vi "Lab Panel V4.83.vi"() -> ()   [LabVIEW 2013] (continued)
                  tunnel: w884 -> [_ w917]
                  tunnel: [w889 w916] -> w883
                  frame False {
                    # "stop test"
                    n577 = stacked-sequence {
                      tunnel: w890 -> [w899 _]
                      tunnel: [w891 _] -> w889
                      frame #0 {
                        n578 = local read "DISP LAB02-2"() -> (w898:T4)
                        n579 = Unbundle(w898) -> ("CYCLE"=w896:dbl, "MINS"=w897:dbl)  [unwired: 1 out]
                        n580 = case shown="\"CYCLE TEST\"" w899 {
                          tunnel: w897 -> [_ _ w906]
                          tunnel: w896 -> [w904 w905 _]
                          tunnel: [w904 w905 w906] -> w895
                          frame "CHART TEST", Default {
                          }
                          frame "CYCLE TEST" {
                          }
                          frame "T-RISE TEST" {
                          }
                        }
                        n581 = local read "TDMS LAB02-2"() -> (w903:refnum<k34>)
                        n582 = Build Array("STOPPED") -> (w900:string[])
                        n583 = Build Array(w895) -> (w894:dbl[])
                        n584 = TDMS Write(0:w903, 5:"TEST RESULT", 7:w900, 9:w894) -> (4:w892:refnum<k34>, 15:w893:errorcluster)  [unwired: 2 in, 2 out]
                        n585 = TDMS Close(8:w893, 11:w892) -> (0:w891:errorcluster)  [unwired: 1 out]
                      }
                      frame #1 {
                        n586 = local read "DISP LAB02-2"() -> (w910:T4)
                        n587 = stacked-sequence {
                          tunnel: "LAB02-2" -> [w912 w914]
                          frame #0 {
                            n588 = call "sub vi - defrag tdms v1.vi"("panel id"=w912) -> ("error out"=w911:errorcluster)  [unwired: 10 in]
                            n589 = local write "data file error"(w911) -> ()
                          }
                          frame #1 {
                            n590 = call "Save data file to network drive v2.vi"("panel id"=w914) -> ("network file save error"=w913:errorcluster)  [unwired: 9 in, 1 out]
                            n591 = local write "RESULT LAB02-2"(FALSE) -> ()
                            n592 = local write "data file error"(w913) -> ()
                          }
                        }
                        n593 = Bundle(cluster=w910, "STATUS"="STOP") -> (w908:T4)  [unwired: 2 in]
                        n594 = local write "DISP LAB02-2"(w908) -> ()
                      }
                    }
                  }
                  frame True {
                    # "start new test and create test file"
                    n595 = stacked-sequence {
                      seq-local: [w922 _ _ _ _] -> [_ w946 _ _ _]
                      tunnel: w921 -> [w927 _ _ _ _]
                      tunnel: w920 -> [w924 _ _ _ _]
                      tunnel: w919 -> [w937 _ _ _ _]
                      tunnel: w918 -> [w930 _ _ _ _]
                      tunnel: w917 -> [w925 _ _ _ _]
                      tunnel: [_ w941 _ _ _] -> w916
                      frame #0 {
                        w923 = "\\"
                        n596 = local read "SET LAB02-2"() -> (w932:T5)
                        n597 = case shown="\"CYCLE TEST\"" w937 {
                          tunnel: ["L02-2-CHART TEST-" "L02-2-CYCLE TEST-" "L02-2-T-RISE TEST-"] -> w933
                          frame "CHART TEST", Default {
                          }
                          frame "CYCLE TEST" {
                          }
                          frame "T-RISE TEST" {
                          }
                        }
                        n598 = Unbundle(w932) -> ("DESCRIPTION"=w931:string)  [unwired: 4 out]
                        n599 = Concatenate Strings(w927, "\\", w925, w923, w924, w923) -> (w934:string)
                        n600 = String To Path(string=w934) -> (path=w936:path)
                        n601 = Concatenate Strings(w934, w933, w931, "-", w930, ".tdms") -> (w922:string)
                        n602 = Create Folder(path (use dialog)=w936) -> (error out=w935:errorcluster)  [unwired: 2 in, 2 out]
                        n603 = global write "Global 1.vi" "LAB02-2 FILE"(w922) -> ()
                        n604 = call <vilib>:"Clear Errors.vi"("error in (no error)"=w935) -> ()  [unwired: 6 in, 1 out]
                      }
                      frame #1 {
                        (unwired) FALSE
                        n605 = String To Path(string=w946) -> (path=w942:path)
                        n606 = TDMS Open(6:FALSE, 10:T18."create or replace" ("operation (0:open)"), 11:w942) -> (0:w941:errorcluster, 3:→"TDMS LAB02-2":refnum<k34>)  [unwired: 4 in]
                      }
                      frame #2 {
                        n607 = local read "SET LAB02-2"() -> (w952:T5)
                        n608 = local read "TDMS LAB02-2"() -> (w963:refnum<k34>)
                        n609 = Build Array("Testers Name", "Description", "Set Test Cycles", "T-Rise minutes", "T-Rise Deg C") -> (w953:string[])
                        n610 = Unbundle(w952) -> ("NAME"=w951:string, "DESCRIPTION"=w950:string, "CYCLES"=w949:dbl, "T-RISE mins"=w948:dbl, "T-RISE deg C"=w947:dbl)
                        n611 = Number To Decimal String(number=w949) -> (decimal integer string=w962:string)  [unwired: 1 in]
                        n612 = Number To Decimal String(number=w948) -> (decimal integer string=w961:string)  [unwired: 1 in]
                        n613 = Number To Decimal String(number=w947) -> (decimal integer string=w960:string)  [unwired: 1 in]
                        n614 = Build Array(w951, w950, w962, w961, w960) -> (w959:string[])
                        n615 = TDMS Set Properties(5:w959, 7:w953, 11:w963) -> ()  [unwired: 3 in, 4 out]
                      }
                      frame #3 {
                        w965 = 0.0
                        n616 = local read "DISP LAB02-2"() -> (w967:T4)
                        n617 = Bundle(cluster=w967, "CYCLE"=w965, "MINS"=w965, "STATUS"="RUN") -> (w966:T4)
                        n618 = local write "DISP LAB02-2"(w966) -> ()
                      }
                      frame #4 {
                        n619 = local read "SIG LAB02-2"() -> (w970:T2)
                        n620 = local read "TEMP START LAB02-2"() -> (w972:cluster{"TL":dbl, "TN":dbl})
                        n621 = Unbundle(w970) -> ("Tmp Live"=w969:dbl, "Tmp Neut"=w968:dbl)  [unwired: 3 out]
                        n622 = Bundle(cluster=w972, "TL"=w969, "TN"=w968) -> (w971:cluster{"TL":dbl, "TN":dbl})
                        n623 = local write "TEMP START LAB02-2"(w971) -> ()
                      }
                    }
                  }
                }
              }
              event "RUN LAB03-1": Value Change {
                n624 = event-data() -> ("NewVal"=w973:bool)  [unwired: 1 in, 5 out]
                n625 = local write "run lab03-1"(w973) -> ()
                n626 = case shown="False" w973 {
                  tunnel: w979 -> [_ w1012]
                  tunnel: w978 -> [_ w1011]
                  tunnel: w976 -> [w981 w1010]
                  tunnel: w977 -> [_ w1009]
                  tunnel: w975 -> [_ w1008]
                  tunnel: [w980 w1007] -> w974
                  frame False {
                    # "stop test"
                    n627 = stacked-sequence {
                      tunnel: w981 -> [w990 _]
                      tunnel: [w982 _] -> w980
                      frame #0 {
                        n628 = local read "DISP LAB03-1"() -> (w989:T4)
                        n629 = Unbundle(w989) -> ("CYCLE"=w987:dbl, "MINS"=w988:dbl)  [unwired: 1 out]
                        n630 = case shown="\"CYCLE TEST\"" w990 {
                          tunnel: w988 -> [_ _ w997]
                          tunnel: w987 -> [w995 w996 _]
                          tunnel: [w995 w996 w997] -> w986
                          frame "CHART TEST", Default {
                          }
                          frame "CYCLE TEST" {
                          }
                          frame "T-RISE TEST" {
                          }
                        }
                        n631 = local read "TDMS LAB03-1"() -> (w994:refnum<k34>)
                        n632 = Build Array("STOPPED") -> (w991:string[])
                        n633 = Build Array(w986) -> (w985:dbl[])
                        n634 = TDMS Write(0:w994, 5:"TEST RESULT", 7:w991, 9:w985) -> (4:w983:refnum<k34>, 15:w984:errorcluster)  [unwired: 2 in, 2 out]
                        n635 = TDMS Close(8:w984, 11:w983) -> (0:w982:errorcluster)  [unwired: 1 out]
                      }
                      frame #1 {
                        n636 = local read "DISP LAB03-1"() -> (w1001:T4)
                        n637 = stacked-sequence {
                          tunnel: "LAB03-1" -> [w1003 w1005]
                          frame #0 {
                            n638 = call "sub vi - defrag tdms v1.vi"("panel id"=w1003) -> ("error out"=w1002:errorcluster)  [unwired: 10 in]
                            n639 = local write "data file error"(w1002) -> ()
                          }
                          frame #1 {
                            n640 = call "Save data file to network drive v2.vi"("panel id"=w1005) -> ("network file save error"=w1004:errorcluster)  [unwired: 9 in, 1 out]
                            n641 = local write "RESULT LAB03-1"(FALSE) -> ()
                            n642 = local write "data file error"(w1004) -> ()
                          }
                        }
                        n643 = Bundle(cluster=w1001, "STATUS"="STOP") -> (w999:T4)  [unwired: 2 in]
                        n644 = local write "DISP LAB03-1"(w999) -> ()
                      }
                    }
                  }
                  frame True {
                    # "start new test and create test file"
                    n645 = stacked-sequence {
                      seq-local: [w1013 _ _ _ _] -> [_ w1037 _ _ _]
                      tunnel: w1012 -> [w1018 _ _ _ _]
                      tunnel: w1011 -> [w1015 _ _ _ _]
                      tunnel: w1010 -> [w1028 _ _ _ _]
                      tunnel: w1009 -> [w1021 _ _ _ _]
                      tunnel: w1008 -> [w1016 _ _ _ _]
                      tunnel: [_ w1032 _ _ _] -> w1007
                      frame #0 {
                        w1014 = "\\"
                        n646 = local read "SET LAB03-1"() -> (w1023:T5)
                        n647 = case shown="\"T-RISE TEST\"" w1028 {
                          tunnel: ["L03-1-CHART TEST-" "L03-1-CYCLE TEST-" "L03-1-T-RISE TEST-"] -> w1024
                          frame "CHART TEST", Default {
                          }
                          frame "CYCLE TEST" {
                          }
                          frame "T-RISE TEST" {
                          }
                        }
                        n648 = Unbundle(w1023) -> ("DESCRIPTION"=w1022:string)  [unwired: 4 out]
                        n649 = Concatenate Strings(w1018, "\\", w1016, w1014, w1015, w1014) -> (w1025:string)
                        n650 = String To Path(string=w1025) -> (path=w1027:path)
                        n651 = Concatenate Strings(w1025, w1024, w1022, "-", w1021, ".tdms") -> (w1013:string)
                        n652 = Create Folder(path (use dialog)=w1027) -> (error out=w1026:errorcluster)  [unwired: 2 in, 2 out]
                        n653 = global write "Global 1.vi" "LAB03-1 FILE"(w1013) -> ()
                        n654 = call <vilib>:"Clear Errors.vi"("error in (no error)"=w1026) -> ()  [unwired: 6 in, 1 out]
                      }
                      frame #1 {
                        (unwired) FALSE
                        n655 = String To Path(string=w1037) -> (path=w1033:path)
                        n656 = TDMS Open(6:FALSE, 10:T18."create or replace" ("operation (0:open)"), 11:w1033) -> (0:w1032:errorcluster, 3:→"TDMS LAB03-1":refnum<k34>)  [unwired: 4 in]
                      }
                      frame #2 {
                        n657 = local read "SET LAB03-1"() -> (w1043:T5)
                        n658 = local read "TDMS LAB03-1"() -> (w1054:refnum<k34>)
                        n659 = Build Array("Testers Name", "Description", "Set Test Cycles", "T-Rise minutes", "T-Rise Deg C") -> (w1044:string[])
                        n660 = Unbundle(w1043) -> ("NAME"=w1042:string, "DESCRIPTION"=w1041:string, "CYCLES"=w1040:dbl, "T-RISE mins"=w1039:dbl, "T-RISE deg C"=w1038:dbl)
                        n661 = Number To Decimal String(number=w1040) -> (decimal integer string=w1053:string)  [unwired: 1 in]
                        n662 = Number To Decimal String(number=w1039) -> (decimal integer string=w1052:string)  [unwired: 1 in]
                        n663 = Number To Decimal String(number=w1038) -> (decimal integer string=w1051:string)  [unwired: 1 in]
                        n664 = Build Array(w1042, w1041, w1053, w1052, w1051) -> (w1050:string[])
                        n665 = TDMS Set Properties(5:w1050, 7:w1044, 11:w1054) -> ()  [unwired: 3 in, 4 out]
                      }
                      frame #3 {
                        w1056 = 0.0
                        n666 = local read "DISP LAB03-1"() -> (w1058:T4)
                        n667 = Bundle(cluster=w1058, "CYCLE"=w1056, "MINS"=w1056, "STATUS"="RUN") -> (w1057:T4)
                        n668 = local write "DISP LAB03-1"(w1057) -> ()
                      }
                      frame #4 {
                        n669 = local read "SIG LAB03-1"() -> (w1061:T2)
                        n670 = local read "TEMP START LAB03-1"() -> (w1063:cluster{"TL":dbl, "TN":dbl})
                        n671 = Unbundle(w1061) -> ("Tmp Live"=w1060:dbl, "Tmp Neut"=w1059:dbl)  [unwired: 3 out]
                        n672 = Bundle(cluster=w1063, "TL"=w1060, "TN"=w1059) -> (w1062:cluster{"TL":dbl, "TN":dbl})
                        n673 = local write "TEMP START LAB03-1"(w1062) -> ()
                      }
                    }
                  }
                }
              }
              event "RUN LAB03-2": Value Change {
                n674 = event-data() -> ("NewVal"=w1064:bool)  [unwired: 1 in, 5 out]
                n675 = local write "run lab03-2"(w1064) -> ()
                n676 = case shown="True" w1064 {
                  tunnel: w1070 -> [_ w1103]
                  tunnel: w1069 -> [_ w1102]
                  tunnel: w1067 -> [w1072 w1101]
                  tunnel: w1068 -> [_ w1100]
                  tunnel: w1066 -> [_ w1099]
                  tunnel: [w1071 w1098] -> w1065
                  frame False {
                    # "stop test"
                    n677 = stacked-sequence {
                      tunnel: w1072 -> [w1081 _]
                      tunnel: [w1073 _] -> w1071
                      frame #0 {
                        n678 = local read "DISP LAB03-2"() -> (w1080:T4)
                        n679 = Unbundle(w1080) -> ("CYCLE"=w1078:dbl, "MINS"=w1079:dbl)  [unwired: 1 out]
                        n680 = case shown="\"CYCLE TEST\"" w1081 {
                          tunnel: w1079 -> [_ _ w1088]
                          tunnel: w1078 -> [w1086 w1087 _]
                          tunnel: [w1086 w1087 w1088] -> w1077
                          frame "CHART TEST", Default {
                          }
                          frame "CYCLE TEST" {
                          }
                          frame "T-RISE TEST" {
                          }
                        }
                        n681 = local read "TDMS LAB03-2"() -> (w1085:refnum<k34>)
                        n682 = Build Array("STOPPED") -> (w1082:string[])
                        n683 = Build Array(w1077) -> (w1076:dbl[])
                        n684 = TDMS Write(0:w1085, 5:"TEST RESULT", 7:w1082, 9:w1076) -> (4:w1074:refnum<k34>, 15:w1075:errorcluster)  [unwired: 2 in, 2 out]
                        n685 = TDMS Close(8:w1075, 11:w1074) -> (0:w1073:errorcluster)  [unwired: 1 out]
                      }
                      frame #1 {
                        n686 = local read "DISP LAB03-2"() -> (w1092:T4)
                        n687 = stacked-sequence {
                          tunnel: "LAB03-2" -> [w1094 w1096]
                          frame #0 {
                            n688 = call "sub vi - defrag tdms v1.vi"("panel id"=w1094) -> ("error out"=w1093:errorcluster)  [unwired: 10 in]
                            n689 = local write "data file error"(w1093) -> ()
                          }
                          frame #1 {
                            n690 = call "Save data file to network drive v2.vi"("panel id"=w1096) -> ("network file save error"=w1095:errorcluster)  [unwired: 9 in, 1 out]
                            n691 = local write "RESULT LAB03-2"(FALSE) -> ()
                            n692 = local write "data file error"(w1095) -> ()
                          }
                        }
                        n693 = Bundle(cluster=w1092, "STATUS"="STOP") -> (w1090:T4)  [unwired: 2 in]
                        n694 = local write "DISP LAB03-2"(w1090) -> ()
                      }
                    }
                  }
                  frame True {
                    # "start new test and create test file"
                    n695 = stacked-sequence {
                      seq-local: [w1104 _ _ _ _] -> [_ w1128 _ _ _]
                      tunnel: w1103 -> [w1109 _ _ _ _]
                      tunnel: w1102 -> [w1106 _ _ _ _]
                      tunnel: w1101 -> [w1119 _ _ _ _]
                      tunnel: w1100 -> [w1112 _ _ _ _]
                      tunnel: w1099 -> [w1107 _ _ _ _]
                      tunnel: [_ w1123 _ _ _] -> w1098
                      frame #0 {
                        w1105 = "\\"
                        n696 = local read "SET LAB03-2"() -> (w1114:T5)
                        n697 = case shown="\"T-RISE TEST\"" w1119 {
                          tunnel: ["L03-2-CHART TEST-" "L03-2-CYCLE TEST-" "L03-2-T-RISE TEST-"] -> w1115
                          frame "CHART TEST", Default {
                          }
                          frame "CYCLE TEST" {
                          }
                          frame "T-RISE TEST" {
                          }
                        }
                        n698 = Unbundle(w1114) -> ("DESCRIPTION"=w1113:string)  [unwired: 4 out]
                        n699 = Concatenate Strings(w1109, "\\", w1107, w1105, w1106, w1105) -> (w1116:string)
                        n700 = String To Path(string=w1116) -> (path=w1118:path)
                        n701 = Concatenate Strings(w1116, w1115, w1113, "-", w1112, ".tdms") -> (w1104:string)
                        n702 = Create Folder(path (use dialog)=w1118) -> (error out=w1117:errorcluster)  [unwired: 2 in, 2 out]
                        n703 = global write "Global 1.vi" "LAB03-2 FILE"(w1104) -> ()
                        n704 = call <vilib>:"Clear Errors.vi"("error in (no error)"=w1117) -> ()  [unwired: 6 in, 1 out]
                      }
                      frame #1 {
                        (unwired) FALSE
                        n705 = String To Path(string=w1128) -> (path=w1124:path)
                        n706 = TDMS Open(6:FALSE, 10:T18."create or replace" ("operation (0:open)"), 11:w1124) -> (0:w1123:errorcluster, 3:→"TDMS LAB03-2":refnum<k34>)  [unwired: 4 in]
                      }
                      frame #2 {
                        n707 = local read "SET LAB03-2"() -> (w1134:T5)
                        n708 = local read "TDMS LAB03-2"() -> (w1145:refnum<k34>)
                        n709 = Build Array("Testers Name", "Description", "Set Test Cycles", "T-Rise minutes", "T-Rise Deg C") -> (w1135:string[])
                        n710 = Unbundle(w1134) -> ("NAME"=w1133:string, "DESCRIPTION"=w1132:string, "CYCLES"=w1131:dbl, "T-RISE mins"=w1130:dbl, "T-RISE deg C"=w1129:dbl)
                        n711 = Number To Decimal String(number=w1131) -> (decimal integer string=w1144:string)  [unwired: 1 in]
                        n712 = Number To Decimal String(number=w1130) -> (decimal integer string=w1143:string)  [unwired: 1 in]
                        n713 = Number To Decimal String(number=w1129) -> (decimal integer string=w1142:string)  [unwired: 1 in]
                        n714 = Build Array(w1133, w1132, w1144, w1143, w1142) -> (w1141:string[])
                        n715 = TDMS Set Properties(5:w1141, 7:w1135, 11:w1145) -> ()  [unwired: 3 in, 4 out]
                      }
                      frame #3 {
                        w1147 = 0.0
                        n716 = local read "DISP LAB03-2"() -> (w1149:T4)
                        n717 = Bundle(cluster=w1149, "CYCLE"=w1147, "MINS"=w1147, "STATUS"="RUN") -> (w1148:T4)
                        n718 = local write "DISP LAB03-2"(w1148) -> ()
                      }
                      frame #4 {
                        n719 = local read "SIG LAB03-2"() -> (w1152:T2)
                        n720 = local read "TEMP START LAB03-2"() -> (w1154:cluster{"TL":dbl, "TN":dbl})
                        n721 = Unbundle(w1152) -> ("Tmp Live"=w1151:dbl, "Tmp Neut"=w1150:dbl)  [unwired: 3 out]
                        n722 = Bundle(cluster=w1154, "TL"=w1151, "TN"=w1150) -> (w1153:cluster{"TL":dbl, "TN":dbl})
                        n723 = local write "TEMP START LAB03-2"(w1153) -> ()
                      }
                    }
                  }
                }
              }
              event "RUN LAB04-1": Value Change {
                n724 = event-data() -> ("NewVal"=w1155:bool)  [unwired: 1 in, 5 out]
                n725 = local write "run lab04-1"(w1155) -> ()
                n726 = case shown="True" w1155 {
                  tunnel: w1161 -> [_ w1194]
                  tunnel: w1160 -> [_ w1193]
                  tunnel: w1158 -> [w1163 w1192]
                  tunnel: w1159 -> [_ w1191]
                  tunnel: w1157 -> [_ w1190]
                  tunnel: [w1162 w1189] -> w1156
                  frame False {
                    # "stop test"
                    n727 = stacked-sequence {
                      tunnel: w1163 -> [w1172 _]
                      tunnel: [w1164 _] -> w1162
                      frame #0 {
                        n728 = local read "DISP LAB04-1"() -> (w1171:T4)
                        n729 = Unbundle(w1171) -> ("CYCLE"=w1169:dbl, "MINS"=w1170:dbl)  [unwired: 1 out]
                        n730 = case shown="\"CYCLE TEST\"" w1172 {
                          tunnel: w1170 -> [_ _ w1179]
                          tunnel: w1169 -> [w1177 w1178 _]
                          tunnel: [w1177 w1178 w1179] -> w1168
                          frame "CHART TEST", Default {
                          }
                          frame "CYCLE TEST" {
                          }
                          frame "T-RISE TEST" {
                          }
                        }
                        n731 = local read "TDMS LAB04-1"() -> (w1176:refnum<k34>)
                        n732 = Build Array("STOPPED") -> (w1173:string[])
                        n733 = Build Array(w1168) -> (w1167:dbl[])
                        n734 = TDMS Write(0:w1176, 5:"TEST RESULT", 7:w1173, 9:w1167) -> (4:w1165:refnum<k34>, 15:w1166:errorcluster)  [unwired: 2 in, 2 out]
                        n735 = TDMS Close(8:w1166, 11:w1165) -> (0:w1164:errorcluster)  [unwired: 1 out]
                      }
                      frame #1 {
                        n736 = local read "DISP LAB04-1"() -> (w1183:T4)
                        n737 = stacked-sequence {
                          tunnel: "LAB04-1" -> [w1185 w1187]
                          frame #0 {
                            n738 = call "sub vi - defrag tdms v1.vi"("panel id"=w1185) -> ("error out"=w1184:errorcluster)  [unwired: 10 in]
                            n739 = local write "data file error"(w1184) -> ()
                          }
                          frame #1 {
                            n740 = call "Save data file to network drive v2.vi"("panel id"=w1187) -> ("network file save error"=w1186:errorcluster)  [unwired: 9 in, 1 out]
                            n741 = local write "RESULT LAB04-1"(FALSE) -> ()
                            n742 = local write "data file error"(w1186) -> ()
                          }
                        }
                        n743 = Bundle(cluster=w1183, "STATUS"="STOP") -> (w1181:T4)  [unwired: 2 in]
                        n744 = local write "DISP LAB04-1"(w1181) -> ()
                      }
                    }
                  }
                  frame True {
                    # "start new test and create test file"
                    n745 = stacked-sequence {
                      seq-local: [w1195 _ _ _ _] -> [_ w1219 _ _ _]
                      tunnel: w1194 -> [w1200 _ _ _ _]
                      tunnel: w1193 -> [w1196 _ _ _ _]
                      tunnel: w1192 -> [w1210 _ _ _ _]
                      tunnel: w1191 -> [w1203 _ _ _ _]
                      tunnel: w1190 -> [w1198 _ _ _ _]
                      tunnel: [_ w1214 _ _ _] -> w1189
                      frame #0 {
                        w1197 = "\\"
                        n746 = local read "SET LAB04-1"() -> (w1205:T5)
                        n747 = case shown="\"CYCLE TEST\"" w1210 {
                          tunnel: ["L04-1-CHART TEST-" "L04-1-CYCLE TEST-" "L04-1-T-RISE TEST-"] -> w1206
                          frame "CHART TEST", Default {
                          }
                          frame "CYCLE TEST" {
                          }
                          frame "T-RISE TEST" {
                          }
                        }
                        n748 = Unbundle(w1205) -> ("DESCRIPTION"=w1204:string)  [unwired: 4 out]
                        n749 = Concatenate Strings(w1200, "\\", w1198, w1197, w1196, w1197) -> (w1207:string)
                        n750 = String To Path(string=w1207) -> (path=w1209:path)
                        n751 = Concatenate Strings(w1207, w1206, w1204, "-", w1203, ".tdms") -> (w1195:string)
                        n752 = Create Folder(path (use dialog)=w1209) -> (error out=w1208:errorcluster)  [unwired: 2 in, 2 out]
                        n753 = global write "Global 1.vi" "LAB04-1 FILE"(w1195) -> ()
                        n754 = call <vilib>:"Clear Errors.vi"("error in (no error)"=w1208) -> ()  [unwired: 6 in, 1 out]
                      }
                      frame #1 {
                        (unwired) FALSE
                        n755 = String To Path(string=w1219) -> (path=w1215:path)
                        n756 = TDMS Open(6:FALSE, 10:T18."create or replace" ("operation (0:open)"), 11:w1215) -> (0:w1214:errorcluster, 3:→"TDMS LAB04-1":refnum<k34>)  [unwired: 4 in]
                      }
                      frame #2 {
                        n757 = local read "SET LAB04-1"() -> (w1225:T5)
                        n758 = local read "TDMS LAB04-1"() -> (w1236:refnum<k34>)
                        n759 = Build Array("Testers Name", "Description", "Set Test Cycles", "T-Rise minutes", "T-Rise Deg C") -> (w1226:string[])
                        n760 = Unbundle(w1225) -> ("NAME"=w1224:string, "DESCRIPTION"=w1223:string, "CYCLES"=w1222:dbl, "T-RISE mins"=w1221:dbl, "T-RISE deg C"=w1220:dbl)
                        n761 = Number To Decimal String(number=w1222) -> (decimal integer string=w1235:string)  [unwired: 1 in]
                        n762 = Number To Decimal String(number=w1221) -> (decimal integer string=w1234:string)  [unwired: 1 in]
                        n763 = Number To Decimal String(number=w1220) -> (decimal integer string=w1233:string)  [unwired: 1 in]
                        n764 = Build Array(w1224, w1223, w1235, w1234, w1233) -> (w1232:string[])
                        n765 = TDMS Set Properties(5:w1232, 7:w1226, 11:w1236) -> ()  [unwired: 3 in, 4 out]
                      }
                      frame #3 {
                        w1238 = 0.0
                        n766 = local read "DISP LAB04-1"() -> (w1240:T4)
                        n767 = Bundle(cluster=w1240, "CYCLE"=w1238, "MINS"=w1238, "STATUS"="RUN") -> (w1239:T4)
                        n768 = local write "DISP LAB04-1"(w1239) -> ()
                      }
                      frame #4 {
                        n769 = local read "SIG LAB04-1"() -> (w1243:T2)
                        n770 = local read "TEMP START LAB04-1"() -> (w1245:cluster{"TL":dbl, "TN":dbl})
                        n771 = Unbundle(w1243) -> ("Tmp Live"=w1242:dbl, "Tmp Neut"=w1241:dbl)  [unwired: 3 out]
                        n772 = Bundle(cluster=w1245, "TL"=w1242, "TN"=w1241) -> (w1244:cluster{"TL":dbl, "TN":dbl})
                        n773 = local write "TEMP START LAB04-1"(w1244) -> ()
                      }
                    }
                  }
                }
              }
              event "RUN LAB04-2": Value Change {
                n774 = event-data() -> ("NewVal"=w1246:bool)  [unwired: 1 in, 5 out]
                n775 = local write "run lab04-2"(w1246) -> ()
                n776 = case shown="True" w1246 {
                  tunnel: w1252 -> [_ w1285]
                  tunnel: w1251 -> [_ w1284]
                  tunnel: w1249 -> [w1254 w1283]
                  tunnel: w1250 -> [_ w1282]
                  tunnel: w1248 -> [_ w1281]
                  tunnel: [w1253 w1280] -> w1247
                  frame False {
                    # "stop test"
                    n777 = stacked-sequence {
                      tunnel: w1254 -> [w1263 _]
                      tunnel: [w1255 _] -> w1253
                      frame #0 {
                        n778 = local read "DISP LAB04-2"() -> (w1262:T4)
                        n779 = Unbundle(w1262) -> ("CYCLE"=w1260:dbl, "MINS"=w1261:dbl)  [unwired: 1 out]
                        n780 = case shown="\"CYCLE TEST\"" w1263 {
                          tunnel: w1261 -> [_ _ w1270]
                          tunnel: w1260 -> [w1268 w1269 _]
                          tunnel: [w1268 w1269 w1270] -> w1259
                          frame "CHART TEST", Default {
                          }
                          frame "CYCLE TEST" {
                          }
                          frame "T-RISE TEST" {
                          }
                        }
                        n781 = local read "TDMS LAB04-2"() -> (w1267:refnum<k34>)
                        n782 = Build Array("STOPPED") -> (w1264:string[])
                        n783 = Build Array(w1259) -> (w1258:dbl[])
                        n784 = TDMS Write(0:w1267, 5:"TEST RESULT", 7:w1264, 9:w1258) -> (4:w1256:refnum<k34>, 15:w1257:errorcluster)  [unwired: 2 in, 2 out]
                        n785 = TDMS Close(8:w1257, 11:w1256) -> (0:w1255:errorcluster)  [unwired: 1 out]
                      }
                      frame #1 {
                        n786 = local read "DISP LAB04-2"() -> (w1274:T4)
                        n787 = stacked-sequence {
                          tunnel: "LAB04-2" -> [w1276 w1278]
                          frame #0 {
                            n788 = call "sub vi - defrag tdms v1.vi"("panel id"=w1276) -> ("error out"=w1275:errorcluster)  [unwired: 10 in]
                            n789 = local write "data file error"(w1275) -> ()
                          }
                          frame #1 {
                            n790 = call "Save data file to network drive v2.vi"("panel id"=w1278) -> ("network file save error"=w1277:errorcluster)  [unwired: 9 in, 1 out]
                            n791 = local write "RESULT LAB04-2"(FALSE) -> ()
                            n792 = local write "data file error"(w1277) -> ()
                          }
                        }
                        n793 = Bundle(cluster=w1274, "STATUS"="STOP") -> (w1272:T4)  [unwired: 2 in]
                        n794 = local write "DISP LAB04-2"(w1272) -> ()
                      }
                    }
                  }
                  frame True {
                    # "start new test and create test file"
                    n795 = stacked-sequence {
                      seq-local: [w1286 _ _ _ _] -> [_ w1310 _ _ _]
                      tunnel: w1285 -> [w1291 _ _ _ _]
                      tunnel: w1284 -> [w1287 _ _ _ _]
                      tunnel: w1283 -> [w1301 _ _ _ _]
                      tunnel: w1282 -> [w1294 _ _ _ _]
                      tunnel: w1281 -> [w1289 _ _ _ _]
                      tunnel: [_ w1305 _ _ _] -> w1280
                      frame #0 {
                        w1288 = "\\"
                        n796 = local read "SET LAB04-2"() -> (w1296:T5)
                        n797 = case shown="\"CHART TEST\", Default" w1301 {
                          tunnel: ["L04-2-CHART TEST-" "L04-2-CYCLE TEST-" "L04-2-T-RISE TEST-"] -> w1297
                          frame "CHART TEST", Default {
                          }
                          frame "CYCLE TEST" {
                          }
                          frame "T-RISE TEST" {
                          }
                        }
                        n798 = Unbundle(w1296) -> ("DESCRIPTION"=w1295:string)  [unwired: 4 out]
                        n799 = Concatenate Strings(w1291, "\\", w1289, w1288, w1287, w1288) -> (w1298:string)
                        n800 = String To Path(string=w1298) -> (path=w1300:path)
                        n801 = Concatenate Strings(w1298, w1297, w1295, "-", w1294, ".tdms") -> (w1286:string)
                        n802 = Create Folder(path (use dialog)=w1300) -> (error out=w1299:errorcluster)  [unwired: 2 in, 2 out]
                        n803 = global write "Global 1.vi" "LAB04-2 FILE"(w1286) -> ()
                        n804 = call <vilib>:"Clear Errors.vi"("error in (no error)"=w1299) -> ()  [unwired: 6 in, 1 out]
                      }
                      frame #1 {
                        (unwired) FALSE
                        n805 = String To Path(string=w1310) -> (path=w1306:path)
                        n806 = TDMS Open(6:FALSE, 10:T18."create or replace" ("operation (0:open)"), 11:w1306) -> (0:w1305:errorcluster, 3:→"TDMS LAB04-2":refnum<k34>)  [unwired: 4 in]
                      }
                      frame #2 {
                        n807 = local read "SET LAB04-2"() -> (w1316:T5)
                        n808 = local read "TDMS LAB04-2"() -> (w1327:refnum<k34>)
                        n809 = Build Array("Testers Name", "Description", "Set Test Cycles", "T-Rise minutes", "T-Rise Deg C") -> (w1317:string[])
                        n810 = Unbundle(w1316) -> ("NAME"=w1315:string, "DESCRIPTION"=w1314:string, "CYCLES"=w1313:dbl, "T-RISE mins"=w1312:dbl, "T-RISE deg C"=w1311:dbl)
                        n811 = Number To Decimal String(number=w1313) -> (decimal integer string=w1326:string)  [unwired: 1 in]
                        n812 = Number To Decimal String(number=w1312) -> (decimal integer string=w1325:string)  [unwired: 1 in]
                        n813 = Number To Decimal String(number=w1311) -> (decimal integer string=w1324:string)  [unwired: 1 in]
                        n814 = Build Array(w1315, w1314, w1326, w1325, w1324) -> (w1323:string[])
                        n815 = TDMS Set Properties(5:w1323, 7:w1317, 11:w1327) -> ()  [unwired: 3 in, 4 out]
                      }
                      frame #3 {
                        w1329 = 0.0
                        n816 = local read "DISP LAB04-2"() -> (w1331:T4)
                        n817 = Bundle(cluster=w1331, "CYCLE"=w1329, "MINS"=w1329, "STATUS"="RUN") -> (w1330:T4)
                        n818 = local write "DISP LAB04-2"(w1330) -> ()
                      }
                      frame #4 {
                        n819 = local read "SIG LAB04-2"() -> (w1334:T2)
                        n820 = local read "TEMP START LAB04-2"() -> (w1336:cluster{"TL":dbl, "TN":dbl})
                        n821 = Unbundle(w1334) -> ("Tmp Live"=w1333:dbl, "Tmp Neut"=w1332:dbl)  [unwired: 3 out]
                        n822 = Bundle(cluster=w1336, "TL"=w1333, "TN"=w1332) -> (w1335:cluster{"TL":dbl, "TN":dbl})
                        n823 = local write "TEMP START LAB04-2"(w1335) -> ()
                      }
                    }
                  }
                }
              }
              event "RUN LAB05-1": Value Change {
                n824 = event-data() -> ("NewVal"=w1337:bool)  [unwired: 1 in, 5 out]
                n825 = local write "run lab05-1"(w1337) -> ()
                n826 = case shown="True" w1337 {
                  tunnel: w1343 -> [_ w1376]
                  tunnel: w1342 -> [_ w1375]
                  tunnel: w1340 -> [w1345 w1374]
                  tunnel: w1341 -> [_ w1373]
                  tunnel: w1339 -> [_ w1372]
                  tunnel: [w1344 w1371] -> w1338
                  frame False {
                    # "stop test"
                    n827 = stacked-sequence {
                      tunnel: w1345 -> [w1354 _]
                      tunnel: [w1346 _] -> w1344
                      frame #0 {
                        n828 = local read "DISP LAB05-1"() -> (w1353:T4)
                        n829 = Unbundle(w1353) -> ("CYCLE"=w1351:dbl, "MINS"=w1352:dbl)  [unwired: 1 out]
                        n830 = case shown="\"CYCLE TEST\"" w1354 {
                          tunnel: w1352 -> [_ _ w1361]
                          tunnel: w1351 -> [w1359 w1360 _]
                          tunnel: [w1359 w1360 w1361] -> w1350
                          frame "CHART TEST", Default {
                          }
                          frame "CYCLE TEST" {
                          }
                          frame "T-RISE TEST" {
                          }
                        }
                        n831 = local read "TDMS LAB05-1"() -> (w1358:refnum<k34>)
                        n832 = Build Array("STOPPED") -> (w1355:string[])
                        n833 = Build Array(w1350) -> (w1349:dbl[])
                        n834 = TDMS Write(0:w1358, 5:"TEST RESULT", 7:w1355, 9:w1349) -> (4:w1347:refnum<k34>, 15:w1348:errorcluster)  [unwired: 2 in, 2 out]
                        n835 = TDMS Close(8:w1348, 11:w1347) -> (0:w1346:errorcluster)  [unwired: 1 out]
                      }
                      frame #1 {
                        n836 = local read "DISP LAB05-1"() -> (w1365:T4)
                        n837 = stacked-sequence {
                          tunnel: "LAB05-1" -> [w1367 w1369]
                          frame #0 {
                            n838 = call "sub vi - defrag tdms v1.vi"("panel id"=w1367) -> ("error out"=w1366:errorcluster)  [unwired: 10 in]
                            n839 = local write "data file error"(w1366) -> ()
                          }
                          frame #1 {
                            n840 = call "Save data file to network drive v2.vi"("panel id"=w1369) -> ("network file save error"=w1368:errorcluster)  [unwired: 9 in, 1 out]
                            n841 = local write "RESULT LAB05-1"(FALSE) -> ()
                            n842 = local write "data file error"(w1368) -> ()
                          }
                        }
                        n843 = Bundle(cluster=w1365, "STATUS"="STOP") -> (w1363:T4)  [unwired: 2 in]
                        n844 = local write "DISP LAB05-1"(w1363) -> ()
                      }
                    }
                  }
                  frame True {
                    # "start new test and create test file"
                    n845 = stacked-sequence {
                      seq-local: [w1377 _ _ _ _] -> [_ w1401 _ _ _]
                      tunnel: w1376 -> [w1382 _ _ _ _]
                      tunnel: w1375 -> [w1378 _ _ _ _]
                      tunnel: w1374 -> [w1392 _ _ _ _]
                      tunnel: w1373 -> [w1385 _ _ _ _]
                      tunnel: w1372 -> [w1380 _ _ _ _]
                      tunnel: [_ w1396 _ _ _] -> w1371
                      frame #0 {
                        w1379 = "\\"
                        n846 = local read "SET LAB05-1"() -> (w1387:T5)
                        n847 = case shown="\"CYCLE TEST\"" w1392 {
                          tunnel: ["L05-1-CHART TEST-" "L05-1-CYCLE TEST-" "L05-1-T-RISE TEST-"] -> w1388
                          frame "CHART TEST", Default {
                          }
                          frame "CYCLE TEST" {
                          }
                          frame "T-RISE TEST" {
                          }
                        }
                        n848 = Unbundle(w1387) -> ("DESCRIPTION"=w1386:string)  [unwired: 4 out]
                        n849 = Concatenate Strings(w1382, "\\", w1380, w1379, w1378, w1379) -> (w1389:string)
                        n850 = String To Path(string=w1389) -> (path=w1391:path)
                        n851 = Concatenate Strings(w1389, w1388, w1386, "-", w1385, ".tdms") -> (w1377:string)
                        n852 = Create Folder(path (use dialog)=w1391) -> (error out=w1390:errorcluster)  [unwired: 2 in, 2 out]
                        n853 = global write "Global 1.vi" "LAB05-1 FILE"(w1377) -> ()
                        n854 = call <vilib>:"Clear Errors.vi"("error in (no error)"=w1390) -> ()  [unwired: 6 in, 1 out]
                      }
                      frame #1 {
                        (unwired) FALSE
                        n855 = String To Path(string=w1401) -> (path=w1397:path)
                        n856 = TDMS Open(6:FALSE, 10:T18."create or replace" ("operation (0:open)"), 11:w1397) -> (0:w1396:errorcluster, 3:→"TDMS LAB05-1":refnum<k34>)  [unwired: 4 in]
                      }
                      frame #2 {
                        n857 = local read "SET LAB05-1"() -> (w1407:T5)
                        n858 = local read "TDMS LAB05-1"() -> (w1418:refnum<k34>)
                        n859 = Build Array("Testers Name", "Description", "Set Test Cycles", "T-Rise minutes", "T-Rise Deg C") -> (w1408:string[])
                        n860 = Unbundle(w1407) -> ("NAME"=w1406:string, "DESCRIPTION"=w1405:string, "CYCLES"=w1404:dbl, "T-RISE mins"=w1403:dbl, "T-RISE deg C"=w1402:dbl)
                        n861 = Number To Decimal String(number=w1404) -> (decimal integer string=w1417:string)  [unwired: 1 in]
                        n862 = Number To Decimal String(number=w1403) -> (decimal integer string=w1416:string)  [unwired: 1 in]
                        n863 = Number To Decimal String(number=w1402) -> (decimal integer string=w1415:string)  [unwired: 1 in]
                        n864 = Build Array(w1406, w1405, w1417, w1416, w1415) -> (w1414:string[])
                        n865 = TDMS Set Properties(5:w1414, 7:w1408, 11:w1418) -> ()  [unwired: 3 in, 4 out]
                      }
                      frame #3 {
                        w1420 = 0.0
                        n866 = local read "DISP LAB05-1"() -> (w1422:T4)
                        n867 = Bundle(cluster=w1422, "CYCLE"=w1420, "MINS"=w1420, "STATUS"="RUN") -> (w1421:T4)
                        n868 = local write "DISP LAB05-1"(w1421) -> ()
                      }
                      frame #4 {
                        n869 = local read "SIG LAB05-1"() -> (w1425:T2)
                        n870 = local read "TEMP START LAB05-1"() -> (w1427:cluster{"TL":dbl, "TN":dbl})
                        n871 = Unbundle(w1425) -> ("Tmp Live"=w1424:dbl, "Tmp Neut"=w1423:dbl)  [unwired: 3 out]
                        n872 = Bundle(cluster=w1427, "TL"=w1424, "TN"=w1423) -> (w1426:cluster{"TL":dbl, "TN":dbl})
                        n873 = local write "TEMP START LAB05-1"(w1426) -> ()
                      }
                    }
                  }
                }
              }
              event "RUN LAB05-2": Value Change {
                n874 = event-data() -> ("NewVal"=w1428:bool)  [unwired: 1 in, 5 out]
                n875 = local write "run lab05-2"(w1428) -> ()
                n876 = case shown="True" w1428 {
                  tunnel: w1434 -> [_ w1467]
                  tunnel: w1433 -> [_ w1466]
                  tunnel: w1431 -> [w1436 w1465]
                  tunnel: w1432 -> [_ w1464]
                  tunnel: w1430 -> [_ w1463]
                  tunnel: [w1435 w1462] -> w1429
                  frame False {
                    # "stop test"
                    n877 = stacked-sequence {
                      tunnel: w1436 -> [w1445 _]
                      tunnel: [w1437 _] -> w1435
                      frame #0 {
                        n878 = local read "DISP LAB05-2"() -> (w1444:T4)
                        n879 = Unbundle(w1444) -> ("CYCLE"=w1442:dbl, "MINS"=w1443:dbl)  [unwired: 1 out]
                        n880 = case shown="\"CYCLE TEST\"" w1445 {
                          tunnel: w1443 -> [_ _ w1452]
                          tunnel: w1442 -> [w1450 w1451 _]
                          tunnel: [w1450 w1451 w1452] -> w1441
                          frame "CHART TEST", Default {
                          }
                          frame "CYCLE TEST" {
                          }
                          frame "T-RISE TEST" {
                          }
                        }
                        n881 = local read "TDMS LAB05-2"() -> (w1449:refnum<k34>)
                        n882 = Build Array("STOPPED") -> (w1446:string[])
                        n883 = Build Array(w1441) -> (w1440:dbl[])
                        n884 = TDMS Write(0:w1449, 5:"TEST RESULT", 7:w1446, 9:w1440) -> (4:w1438:refnum<k34>, 15:w1439:errorcluster)  [unwired: 2 in, 2 out]
                        n885 = TDMS Close(8:w1439, 11:w1438) -> (0:w1437:errorcluster)  [unwired: 1 out]
                      }
                      frame #1 {
                        n886 = local read "DISP LAB05-2"() -> (w1456:T4)
                        n887 = stacked-sequence {
                          tunnel: "LAB05-2" -> [w1458 w1460]
                          frame #0 {
                            n888 = call "sub vi - defrag tdms v1.vi"("panel id"=w1458) -> ("error out"=w1457:errorcluster)  [unwired: 10 in]
                            n889 = local write "data file error"(w1457) -> ()
                          }
                          frame #1 {
                            n890 = local write "RESULT LAB05-2"(FALSE) -> ()
                            n891 = call "Save data file to network drive v2.vi"("panel id"=w1460) -> ("network file save error"=w1459:errorcluster)  [unwired: 9 in, 1 out]
                            n892 = local write "data file error"(w1459) -> ()
                          }
                        }
                        n893 = Bundle(cluster=w1456, "STATUS"="STOP") -> (w1454:T4)  [unwired: 2 in]
                        n894 = local write "DISP LAB05-2"(w1454) -> ()
                      }
                    }
                  }
                  frame True {
                    # "start new test and create test file"
                    n895 = stacked-sequence {
                      seq-local: [w1468 _ _ _ _] -> [_ w1492 _ _ _]
                      tunnel: w1467 -> [w1473 _ _ _ _]
                      tunnel: w1466 -> [w1469 _ _ _ _]
                      tunnel: w1465 -> [w1483 _ _ _ _]
                      tunnel: w1464 -> [w1476 _ _ _ _]
                      tunnel: w1463 -> [w1471 _ _ _ _]
                      tunnel: [_ w1487 _ _ _] -> w1462
                      frame #0 {
                        w1470 = "\\"
                        n896 = local read "SET LAB05-2"() -> (w1478:T5)
                        n897 = case shown="\"CYCLE TEST\"" w1483 {
                          tunnel: ["L05-2-CHART TEST-" "L05-2-CYCLE TEST-" "L05-2-T-RISE TEST-"] -> w1479
                          frame "CHART TEST", Default {
                          }
                          frame "CYCLE TEST" {
                          }
                          frame "T-RISE TEST" {
                          }
                        }
                        n898 = Unbundle(w1478) -> ("DESCRIPTION"=w1477:string)  [unwired: 4 out]
                        n899 = Concatenate Strings(w1473, "\\", w1471, w1470, w1469, w1470) -> (w1480:string)
                        n900 = String To Path(string=w1480) -> (path=w1482:path)
                        n901 = Concatenate Strings(w1480, w1479, w1477, "-", w1476, ".tdms") -> (w1468:string)
                        n902 = Create Folder(path (use dialog)=w1482) -> (error out=w1481:errorcluster)  [unwired: 2 in, 2 out]
                        n903 = global write "Global 1.vi" "LAB05-2 FILE"(w1468) -> ()
                        n904 = call <vilib>:"Clear Errors.vi"("error in (no error)"=w1481) -> ()  [unwired: 6 in, 1 out]
                      }
                      frame #1 {
                        (unwired) FALSE
                        n905 = String To Path(string=w1492) -> (path=w1488:path)
